vi "add_peak_center_data.vi"(8 "error in (no error)":errorcluster, 10 "peakcenter data":string[](array[string]), 11 "Analysis in":refnum<class "Analysis.lvclass">) -> (0 "error out":errorcluster, 3 "Analysis out":refnum<class "Analysis.lvclass">)   [LabVIEW 2018, in "Analysis.lvclass"]
doc: "ads the peal center data to the peak center array\nisoope_name, magnet_value"
uses:
  Analysis.lvclass
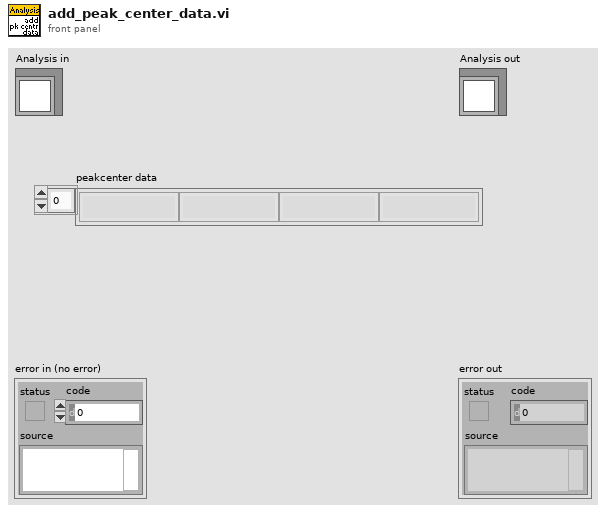
[diagram p1: front panel]
types:
  T1 = typedef "PeakCenterArray.ctl" = string[][]
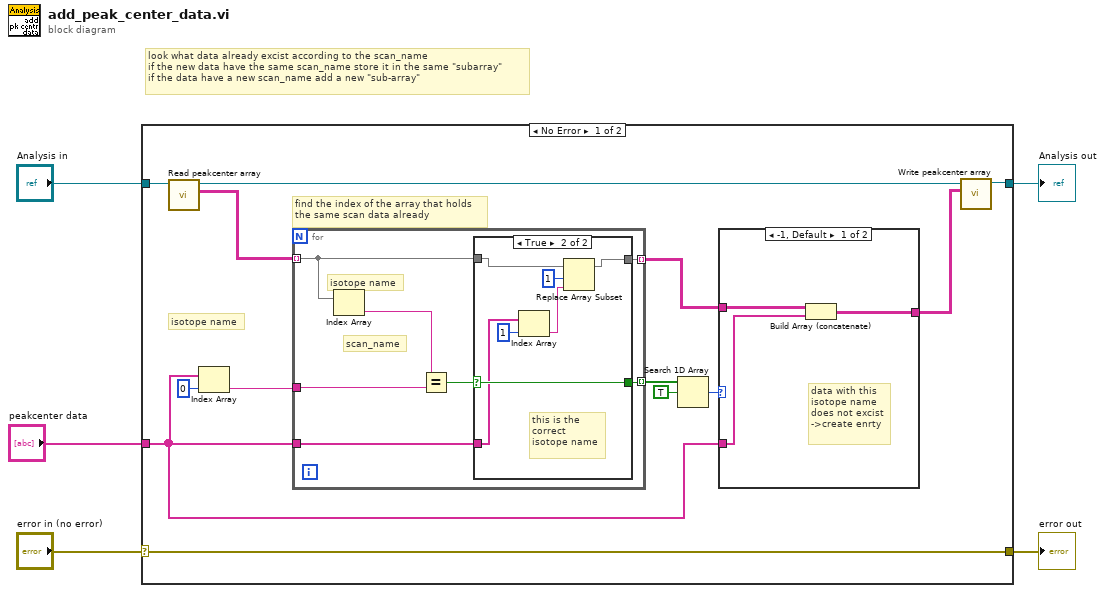
[diagram p0: block diagram]
diagram:
  # "look what data already excist according to the scan_name\nif the new data have the same scan_name store it in the same \"subarray\"\nif the data have a new scan_name add a new \"sub-array\""
  n1 = case shown="No Error" "error in (no error)" {
    selector: "error in (no error)" -> [w18 w40]
    tunnel: [w18 w40] -> w4
    tunnel: [w15 w39] -> w2
    tunnel: "Analysis in" -> [w17 w39]
    tunnel: "peakcenter data" -> [w6 _]
    frame No Error {
      # "find the index of the array that holds\nthe same scan data already"
      # "isotope name"
      n2 = call-dynamic "Read peakcenter array.vi"("Analysis in"=w17) -> ("peakcenter array"=w13:T1, "Analysis out"=w16:refnum<class "Analysis.lvclass">)  [unwired: 8 in, 1 out]
      n3 = Index Array(array=w6, index=0) -> (element=w11:string)
      n4 = for {
        tunnel: w13 -> [w25] mode=indexing
        tunnel: w11 -> [w29]
        tunnel: [w26] -> w12 mode=indexing
        tunnel: [w24] -> w8 mode=indexing
        tunnel: w6 -> [w28]
        # "scan_name"
        # "isotope name"
        n5 = Index Array(array=w25) -> (element=w23:string)  [unwired: 1 in]
        n6 = Equal?(x=w23, y=w29) -> (x = y?=w27:bool)
        n7 = case shown="True" w27 {
          selector: w27 -> [w31 w38]
          tunnel: w28 -> [_ w34]
          tunnel: [w31 w38] -> w26
          tunnel: w25 -> [w30 w37]
          tunnel: [w30 w36] -> w24
          frame False {
            # "not the right\nsub-array"
          }
          frame True {
            # "this is the\ncorrect\nisotope name"
            n8 = Index Array(array=w34, index=1) -> (element=w32:string)
            n9 = Replace Array Subset(array=w37, new element=w32, index=1) -> (w36:string[])
          }
        }
      }
      n10 = Search 1D Array(1D array=w12, element=TRUE) -> (index of element=w9:i32)  [unwired: 1 in]
      n11 = case shown="-1, Default" w9 {
        tunnel: w8 -> [w20 w22]
        tunnel: w6 -> [w19 _]
        tunnel: [w21 w22] -> w7
        frame -1, Default {
          # "data with this\nisotope name\ndoes not excist\n->create enrty"
          n12 = Build Array (concatenate)(w20, w19) -> (w21:string[][])
        }
        frame 0.. {
          # "all fine, data have been\ninserted already"
        }
      }
      n13 = call-dynamic "Write peakcenter array.vi"("peakcenter array"=w7, "Analysis in"=w16) -> ("Analysis out"=w15:refnum<class "Analysis.lvclass">)  [unwired: 8 in, 1 out]
    }
    frame Error {
    }
  }
  "error out" <- w4
  "Analysis out" <- w2
